vi "citTemplate.writeQueue.vi"(1 "High priority (F)":bool, 2 "instance (0)":i32, 5 "event in (if not connected:all statemachine with data event)":variant, 9 "data in":string, 11 "error in (no error)":errorcluster) -> (15 "error out":errorcluster)   [LabVIEW 2019, in "Tools.lvlib"]
uses:
  Tools.lvlib
  citTemplate.notifierHandle.ctl
  citTemplate.notifierData.ctl
  citTemplate.eventQueue.ctl
panel:
  in  "Event data":T2
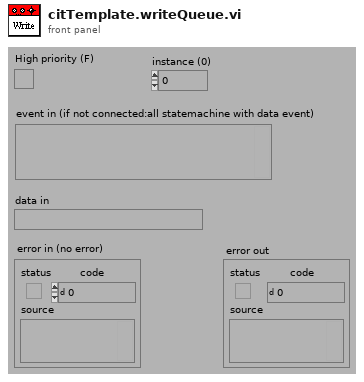
[diagram p1: front panel]
types:
  T1 = typedef "Tools.lvlib/citTemplate.notifierHandle.ctl" = refnum<notifier>
  T2 = cluster{"event index":u32, "(flatten) data in":string, "ack notifier":T1}
  T3 = typedef "Tools.lvlib/citTemplate.eventQueue.ctl" = enum16{"create queue", "get queue handle(s)", "destroy queue"}
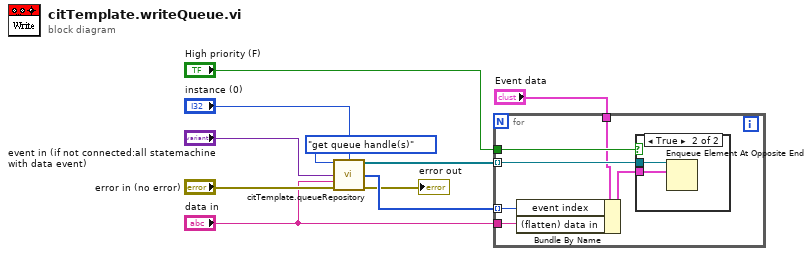
[diagram p0: block diagram]
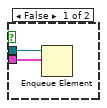
[diagram p2: hidden frame]
diagram:
  n1 = call "citTemplate.queueRepository.vi"("mode (get queue handle)"=citTemplate.eventQueue."get queue handle(s)" ("mode (write event)"), "instance (0)"="instance (0)", "event in"="event in (if not connected:all statemachine with data event)", "(flatten) data in"="data in", "error in (no error)"="error in (no error)") -> ("queueHandle(s) out"=w8:refnum<queue>[], "eventIndex(s)"=w4:u32[], "error out"=→"error out":errorcluster)  [unwired: 1 in, 7 out]
  n2 = for {
    tunnel: w8 -> [w16] mode=indexing
    tunnel: "High priority (F)" -> [w15]
    tunnel: "data in" -> [w14]
    tunnel: w4 -> [w13] mode=indexing
    tunnel: "Event data" -> [w12]
    n3 = Bundle By Name(cluster=w12, "event index"=w13, "(flatten) data in"=w14) -> (w11:T2)
    n4 = case shown="True" w15 {
      tunnel: w16 -> [w18 w20]
      tunnel: w11 -> [w17 w19]
      frame False {
        n5 = Enqueue Element(queue=w18, element=w17) -> ()  [unwired: 1 in, 4 out]
      }
      frame True {
        n6 = Enqueue Element At Opposite End(queue=w20, element=w19) -> ()  [unwired: 1 in, 4 out]
      }
    }
  }
